vi "Update Graphs.vi"(8 "error in (no error)":errorcluster, 11 "Sensor & Control in":refnum<class "Sensor & Control.lvclass">) -> (0 "error out":errorcluster, 3 "Sensor & Control out":refnum<class "Sensor & Control.lvclass">)   [LabVIEW 2013, in "Sensor & Control.lvlib" / "Sensor & Control.lvclass"]
uses:
  Sensor & Control.lvclass
  Sensor & Control.lvclass/Sensor & Control.ctl
  Read Graph History.vi
  Read Graph.vi
  PluginInterface/PluginInterface.lvlibp/PluginInterfaceClass/Read Name.vi
  PluginInterface/PluginInterface.lvlibp/PluginInterfaceClass/Read TDMS.vi
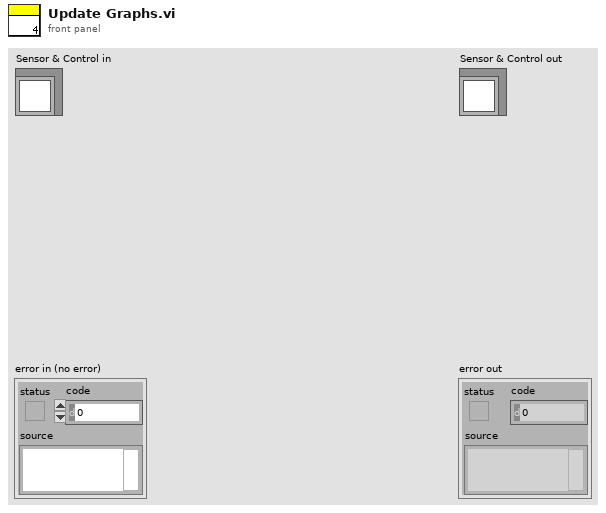
[diagram p1: front panel]
types:
  T1 = cluster{"output array":dbl[], "output array":dbl[]}
  T2 = cluster{"output array":dbl[], "output array":dbl[]}[]
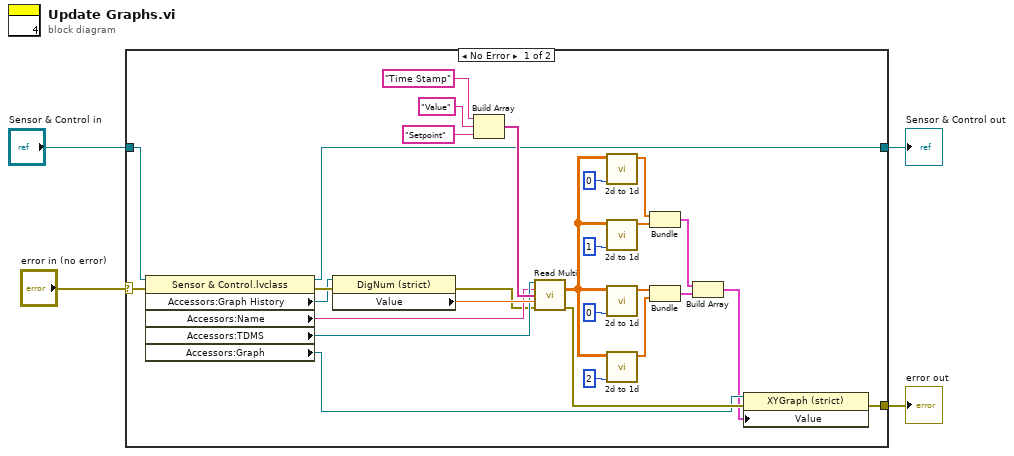
[diagram p0: block diagram]
diagram:
  n1 = case shown="No Error" "error in (no error)" {
    selector: "error in (no error)" -> [w28 w34]
    tunnel: [w8 w34] -> w1
    tunnel: [w5 w33] -> w2
    tunnel: "Sensor & Control in" -> [w32 w33]
    frame No Error {
      n2 = property class="Sensor & Control.lvclass"(reference=w32, error in=w28) -> (reference out=w5:refnum<class "Sensor & Control.lvclass">, error out=w27:errorcluster, "Accessors:Graph History"=w23:refnum<vi>, "Accessors:Name"=w7:string, "Accessors:TDMS"=w24:refnum<k34>, "Accessors:Graph"=w21:refnum<vi>)
      n3 = property class="DigNum (strict)"(reference=w23, error in=w27) -> (error out=w6:errorcluster, "Value"=w25:dbl)  [unwired: 1 out]
      n4 = Build Array("Time Stamp" ("Channel"), "Value" ("string"), "Setpoint" ("string")) -> (w26:string[])
      n5 = call "Read Multi.vi"("tdms file in"=w24, "group"=w7, "Channel"=w26, "Numeric"=w25, "error in (no error)"=w6) -> ("Array"=w12:dbl[][], "error out"=w22:errorcluster)  [unwired: 7 in, 2 out]
      n6 = call "2d to 1d.vi"("index"=0, "array"=w12) -> ("output array"=w15:dbl[])  [unwired: 9 in]
      n7 = call "2d to 1d.vi"("index"=1, "array"=w12) -> ("output array"=w10:dbl[])  [unwired: 9 in]
      n8 = call "2d to 1d.vi"("index"=0, "array"=w12) -> ("output array"=w16:dbl[])  [unwired: 9 in]
      n9 = call "2d to 1d.vi"("index"=2, "array"=w12) -> ("output array"=w9:dbl[])  [unwired: 9 in]
      n10 = Bundle("output array"=w15, "output array"=w10) -> (w14:T1)  [unwired: 1 in]
      n11 = Bundle("output array"=w16, "output array"=w9) -> (w13:T1)  [unwired: 1 in]
      n12 = Build Array(w14, w13) -> (w11:T2)
      n13 = property class="XYGraph (strict)"(reference=w21, error in=w22, "Value"=w11) -> (error out=w8:errorcluster)  [unwired: 1 out]
    }
    frame Error {
    }
  }
  "error out" <- w1
  "Sensor & Control out" <- w2
